vi "add_param.vi"(5 "name":string, 7 "value":string, 8 "error in (no error)":errorcluster, 10 "parent element in":refnum<class "XMLElement.lvclass">, 11 "SoftwareParameter in":refnum<class "SoftwareParameter.lvclass">) -> (0 "error out":errorcluster, 2 "parent element out":refnum<class "XMLElement.lvclass">, 3 "SoftwareParameter out":refnum<class "SoftwareParameter.lvclass">)   [LabVIEW 2010, in "SoftwareParameter.lvclass"]
uses:
  SoftwareParameter.lvclass
  XMLElement/XMLElement/XMLElement.lvclass
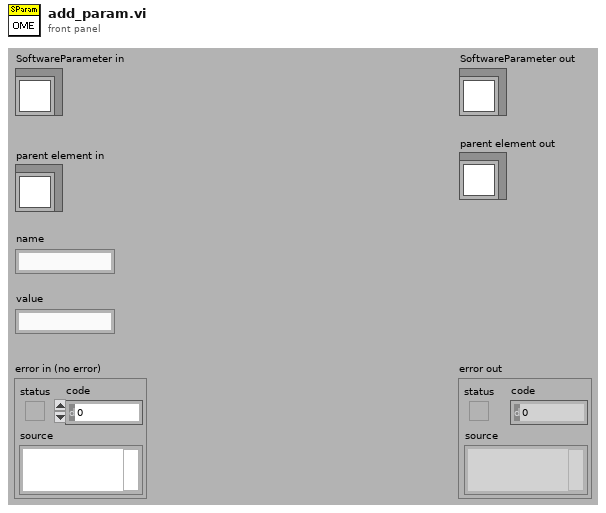
[diagram p1: front panel]
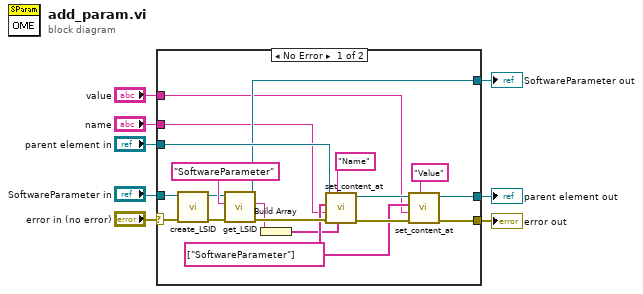
[diagram p0: block diagram]
diagram:
  n1 = case shown="No Error" "error in (no error)" {
    selector: "error in (no error)" -> [w16 w30]
    tunnel: "parent element in" -> [w25 w29]
    tunnel: "SoftwareParameter in" -> [w14 w28]
    tunnel: "name" -> [w12 _]
    tunnel: "value" -> [w13 _]
    tunnel: [w22 w30] -> w3
    tunnel: [w21 w29] -> w2
    tunnel: [w20 w28] -> w1
    frame No Error {
      w18 = string[] ["SoftwareParameter"]
      n2 = call-dynamic "create_LSID.vi"("error in (no error)"=w16, "GenericPlugin in"=w14) -> ("error out"=w17:errorcluster, "GenericPlugin out"=w15:refnum<class "SoftwareParameter.lvclass">)  [unwired: 7 in, 1 out]
      n3 = call-dynamic "get_LSID.vi"("error in (no error)"=w17, "namespace"="SoftwareParameter", "GenericPlugin in"=w15) -> ("error out"=w26:errorcluster, "LSID (string)"=w19:string, "GenericPlugin out"=w20:refnum<class "SoftwareParameter.lvclass">)  [unwired: 5 in, 1 out]
      n4 = Build Array(w19) -> (w10:string[])
      n5 = call "set_content_at.vi"("id chain"=w10, "attribute name"="Name", "error in (no error)"=w26, "content"=w12, "key chain"=w18, "Element in"=w25) -> ("error out"=w24:errorcluster, "Element out"=w23:refnum<class "XMLElement.lvclass">)  [unwired: 4 in]
      n6 = call "set_content_at.vi"("attribute name"="Value", "error in (no error)"=w24, "content"=w13, "key chain"=w18, "Element in"=w23) -> ("error out"=w22:errorcluster, "Element out"=w21:refnum<class "XMLElement.lvclass">)  [unwired: 5 in]
    }
    frame Error {
    }
  }
  "error out" <- w3
  "SoftwareParameter out" <- w1
  "parent element out" <- w2
